vi "Interpolate Points (Distance).vi"(1 "End Point":cluster{"X":dbl, "Y":dbl}, 2 "Distance between Points":dbl, 3 "Start Point":cluster{"X":dbl, "Y":dbl}) -> (0 "Output Point Array":cluster{"X":dbl, "Y":dbl}[](array[cluster]))   [LabVIEW 2020]
doc: "This VI interpolates at specified intervals between two points."
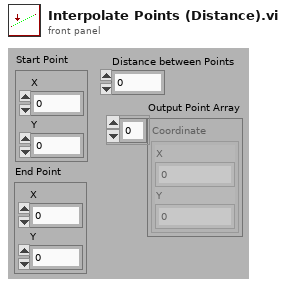
[diagram p1: front panel]
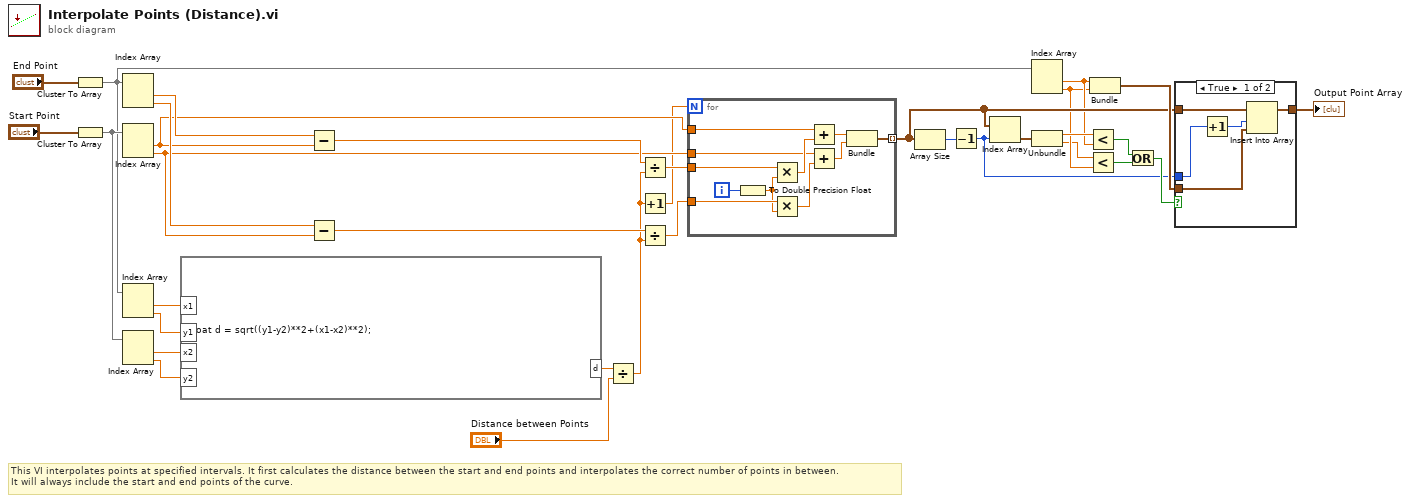
[diagram p0: block diagram]
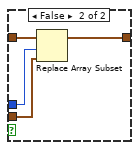
[diagram p2: hidden frame]
diagram:
  # "This VI interpolates points at specified intervals. It first calculates the distance between the start and end points and interpolates the correct number of points in between. \nIt will always include the start and end points of the curve."
  n1 = Cluster To Array(cluster="End Point") -> (array=w13:dbl[])
  n2 = Cluster To Array(cluster="Start Point") -> (array=w14:dbl[])
  n3 = Index Array(array=w13) -> (element #1=w33:dbl, element #2=w30:dbl)  [unwired: 2 in]
  n4 = Index Array(array=w14) -> (element #1=w29:dbl, element #2=w27:dbl)  [unwired: 2 in]
  n5 = Index Array(array=w13) -> (element #1=w22:dbl, element #2=w21:dbl)  [unwired: 2 in]
  n6 = Index Array(array=w14) -> (element #1=w24:dbl, element #2=w23:dbl)  [unwired: 2 in]
  n7 = formula code="float d = sqrt((y1-y2)**2+(x1-x2)**2);"("x1"=w22, "y1"=w21, "x2"=w24, "y2"=w23) -> ("d"=w20:dbl)
  n8 = Subtract(x=w33, y=w29) -> (x-y=w32:dbl)
  n9 = Subtract(x=w30, y=w27) -> (x-y=w31:dbl)
  n10 = Divide(x=w20, y="Distance between Points") -> (x/y=w18:dbl)
  n11 = Divide(x=w32, y=w18) -> (x/y=w28:dbl)
  n12 = Increment(x=w18) -> (x+1=w25:dbl)
  n13 = Divide(x=w31, y=w18) -> (x/y=w26:dbl)
  n14 = for {
    N: w25 -> [_]
    tunnel: w29 -> [w44]
    tunnel: w28 -> [w43]
    tunnel: w27 -> [w41]
    tunnel: w26 -> [w40]
    tunnel: [w36] -> w7 mode=indexing
    i -> [w35]
    n15 = To Double Precision Float(number=w35) -> (double precision float=w34:dbl)
    n16 = Multiply(x=w43, y=w34) -> (x*y=w42:dbl)
    n17 = Multiply(x=w40, y=w34) -> (x*y=w39:dbl)
    n18 = Add(x=w44, y=w42) -> (x+y=w38:dbl)
    n19 = Add(x=w41, y=w39) -> (x+y=w37:dbl)
    n20 = Bundle(w38, w37) -> (w36:cluster{dbl, dbl})  [unwired: 1 out]
  }
  n21 = Array Size(array=w7) -> (size(s)=w16:i32)
  n22 = Decrement(x=w16) -> (x-1=w6:i32)
  n23 = Index Array(array=w7, index=w6) -> (element=w5:cluster{dbl, dbl})
  n24 = Index Array(array=w13) -> (element #1=w3:dbl, element #2=w2:dbl)  [unwired: 2 in]
  n25 = Unbundle(w5) -> (w4:dbl, w1:dbl)
  n26 = Less?(x=w4, y=w3) -> (x < y?=w9:bool)
  n27 = Less?(x=w1, y=w2) -> (x < y?=w10:bool)
  n28 = Bundle("X"=w3, "X"=w2) -> (w17:cluster{"X":dbl, "X":dbl})  [unwired: 1 in]
  n29 = Or(x=w9, y=w10) -> (x .or. y?=w8:bool)
  n30 = case shown="True" w8 {
    tunnel: w7 -> [w49 w53]
    tunnel: w17 -> [w48 w52]
    tunnel: w6 -> [w46 w51]
    tunnel: [w47 w50] -> w11
    frame True {
      n31 = Increment(x=w46) -> (x+1=w45:i32)
      n32 = Insert Into Array(array=w49, index=w45, new element=w48) -> (w47:cluster{dbl, dbl}[])
    }
    frame False {
      n33 = Replace Array Subset(array=w53, new element=w52, index=w51) -> (w50:cluster{dbl, dbl}[])
    }
  }
  "Output Point Array" <- w11
